vi "execute_tango_archive.vi"(10 "Data Name":string, 11 "Numeric":dbl) -> (0 "error out":errorcluster)   [LabVIEW 2020]
uses:
  <vilib>/LabVIEW Open Source Project/Epoch Date & Time/epoch.UNIX/Epoch.UNIX.lvclass
  C:/Program Files (x86)/National Instruments/LabVIEW 2020/vi.lib/LabVIEW Open Source Project/Epoch Date & Time/epoch/Epoch.lvclass
  <vilib>/LabVIEW Open Source Project/Epoch Date & Time/Get Epoch Time.vi
  tango-binding-3.0.0-for-labview-2015-windows-x86/vis/tango_vi.llb/fromDevString.vi
  <vilib>/addons/Tools/Unicode/UTF8 Tools.lvlib
  tango-binding-3.0.0-for-labview-2015-windows-x86/vis/tango_vi.llb/tango.lvlib
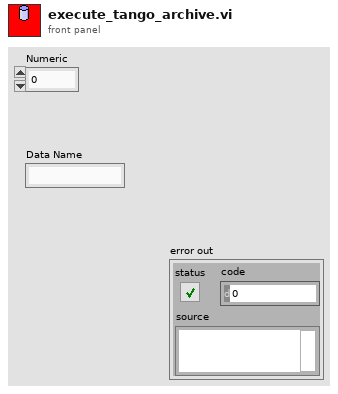
[diagram p1: front panel]
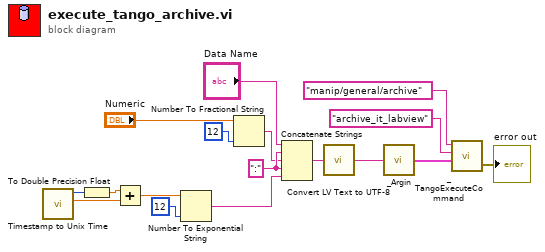
[diagram p0: block diagram]
diagram:
  w10 = ":" ("string")
  n1 = call <vilib>:"Timestamp to Unix Time.vi"() -> ("Fractional Second"=w17:dbl, "Unix Time (s)"=w16:i64)  [unwired: 10 in]
  n2 = To Double Precision Float(number=w16) -> (double precision float=w11:dbl)
  n3 = Add(x=w11, y=w17) -> (x+y=w13:dbl)
  n4 = Number To Exponential String(number=w13, precision (6)=i16 12) -> (E-format string=w14:string)  [unwired: 2 in]
  n5 = Number To Fractional String(number="Numeric", precision (6)=i16 12) -> (F-format string=w2:string)  [unwired: 2 in]
  n6 = Concatenate Strings("Data Name", w10, w2, w10, w14) -> (w5:string)
  n7 = call <vilib>:"Convert LV Text to UTF-8.vi"("LV Text"=w5) -> ("UTF-8 Text"=w9:string)  [unwired: 13 in, 1 out]
  n8 = call-poly "_Argin.vi"("argin"=w9) -> ("ArgIO"=w8:cluster{"num data":u8[], "str data":string[]})
  n9 = call "_TangoExecuteCommand.vi"("argin"=w8, "command name"="archive_it_labview" ("device name"), "device name"="manip/general/archive" ("command name")) -> ("error out"=→"error out":errorcluster)  [unwired: 1 in, 1 out]
